vi "Error Constants.vi"() -> ()   [LabVIEW 2025, in "Runtime Configuration Support Inline Async Example System Explorer.lvlib"]
uses:
  Runtime Configuration Support Inline Async Example System Explorer.lvlib
panel:
  in  "Tab Control":enum32{"Constants"}(tab)
  in  "Error_MissingSignalID":string="The property 'SignalID' is missing in one or more dynamically configured channels. Each channel must have a 'SignalID' property."
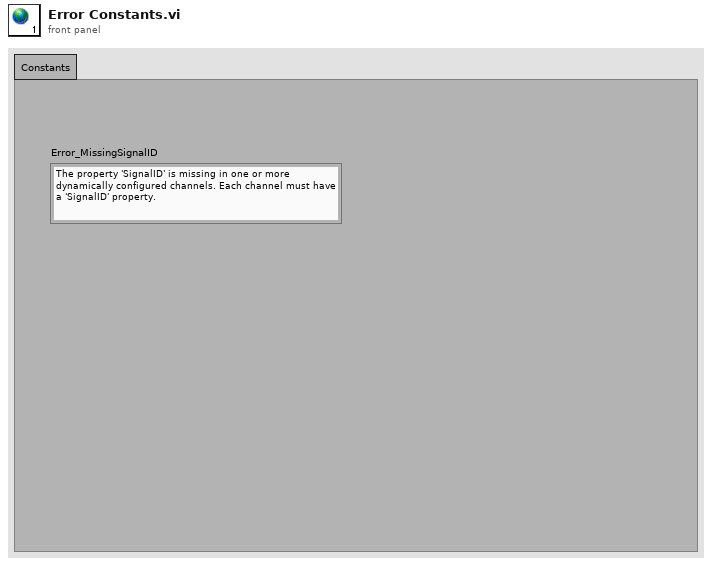
[diagram p1: front panel]
diagram:
